vi "enumerateStaticDependencies.vi"(8 "error in (no error)":errorcluster, 11 "Instrument.Lockin":refnum<class "Instrument.Lockin.lvclass">) -> (0 "error out":errorcluster, 2 "Static Dependencies":refnum<class "Dependency.lvclass">[](array[class]), 3 "Instrument.Lockin out":refnum<class "Instrument.Lockin.lvclass">)   [LabVIEW 2019, in "Instrument.Lockin.lvlib" / "Instrument.Lockin.lvclass"]
doc: "JKI State Machine Objects (SMO) 1.3.0.56\nJKI - JKI\nCopyright (c) 2017, JKI"
uses:
  Instrument.Lockin.lvclass
  <vilib>/JKI/JKI SMO/Dependency/Dependency.lvclass
  Instrument.Lockin.lvclass/Instrument.Lockin.ctl
  Instrument.DAQ/Instrument.DAQ.lvclass
  C:/Program Files/National Instruments/LabVIEW 2019/vi.lib/JKI/JKI SMO/SMO/SMO.lvclass
  <userlib>/LevyLab/Instrument Framework/Instrument Types/Lockin/Instrument.LockinAPI.lvclass
  <vilib>/JKI/JKI SMO/SMO/SMO.lvclass
panel:
  # "For instructions on how to use the JKI State Machine Objects, examples and video tutorials, visit:\nhttp://jki.net/state-machine-objects/\n\nJKI State Machine Objects™\nhttp://jki.net/state-machine-objects/\nCopyright (C) 2005-2015, JKI <info@jki.net>\nALL RIGHTS RESERVED"
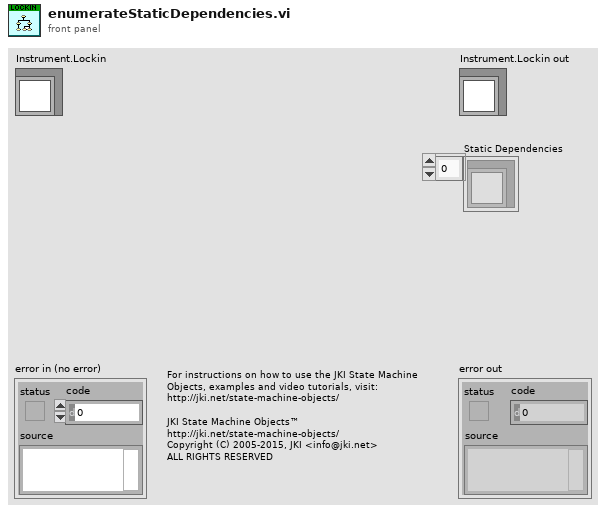
[diagram p1: front panel]
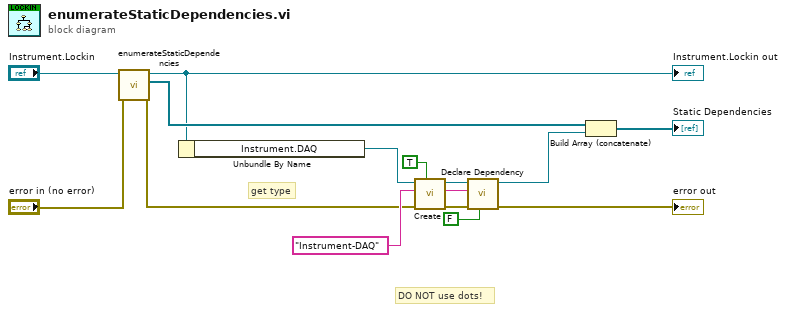
[diagram p0: block diagram]
diagram:
  # "get type"
  # "DO NOT use dots!"
  n1 = call-parent "enumerateStaticDependencies.vi"("error in (no error)"="error in (no error)", "Instrument"="Instrument.Lockin") -> ("error out"=w12:errorcluster, "Static Dependencies"=w11:refnum<class "Dependency.lvclass">[], "Instrument out"=w8:refnum<class "Instrument.Lockin.lvclass">)  [unwired: 7 in]
  "Instrument.Lockin out" <- w8
  n2 = Unbundle By Name(w8) -> ("Instrument.DAQ"=w10:refnum<class "Instrument.DAQ.lvclass">)
  n3 = call <vilib>:"Create.vi"("Shared Resource (F)"=TRUE, "error in (no error)"=w12, "Subsystem Name (optional)"="Instrument-DAQ" ("Name"), "SMO"=w10) -> ("error out"=w6:errorcluster, "SMO name"=w5:string, "SMO out"=w7:refnum<class "Instrument.DAQ.lvclass">)  [unwired: 5 in]
  n4 = call <vilib>:"Declare Dependency.vi"("Shared Resource (F)"=FALSE, "error in (no error)"=w6, "Name"=w5, "Type"=w7) -> ("error out"=→"error out":errorcluster, "Dependency out"=w4:refnum<class "Dependency.lvclass">)  [unwired: 6 in]
  n5 = Build Array (concatenate)(w11, w4) -> (→"Static Dependencies":refnum<class "Dependency.lvclass">[])
